vi "fgv_pc_clamp_result.vi"(7 "cmd":T6=enum."write_clamp_result", 8 "error in":errorcluster, 9 "clamp_roi_overlay-result_in":T3 {"ROI Descriptor out"."Contours"."Type" items=["No Selection", "Point", "Line", "Rectangle", "Oval", "Polygon", "Freehand Region", "Annulus", "Unused2", "Unused3", "Broken Line", "Freehand Line", "Rotated Rectangle"]}, 10 "mask_sum":cluster{u8, u8}, 11 "clamp result in":T5 {"clamp_result"."ROI Descriptor out"."Contours"."Type" items=["No Selection", "Point", "Line", "Rectangle", "Oval", "Polygon", "Freehand Region", "Annulus", "Unused2", "Unused3", "Broken Line", "Freehand Line", "Rotated Rectangle"]}) -> (0 "error out":errorcluster, 1 "clamp_roi_overlay-result_out":T2 {"ROI Descriptor out"."Contours"."Type" items=["No Selection", "Point", "Line", "Rectangle", "Oval", "Polygon", "Freehand Region", "Annulus", "Unused2", "Unused3", "Broken Line", "Freehand Line", "Rotated Rectangle"]}, 2 "mask_sum_out":cluster{u8, u8}, 3 "clamp result out":T4 {"clamp_result"."ROI Descriptor out"."Contours"."Type" items=["No Selection", "Point", "Line", "Rectangle", "Oval", "Polygon", "Freehand Region", "Annulus", "Unused2", "Unused3", "Broken Line", "Freehand Line", "Rotated Rectangle"]})   [LabVIEW 2019]
uses:
  Ctrl/clamp-result_cmd.ctl
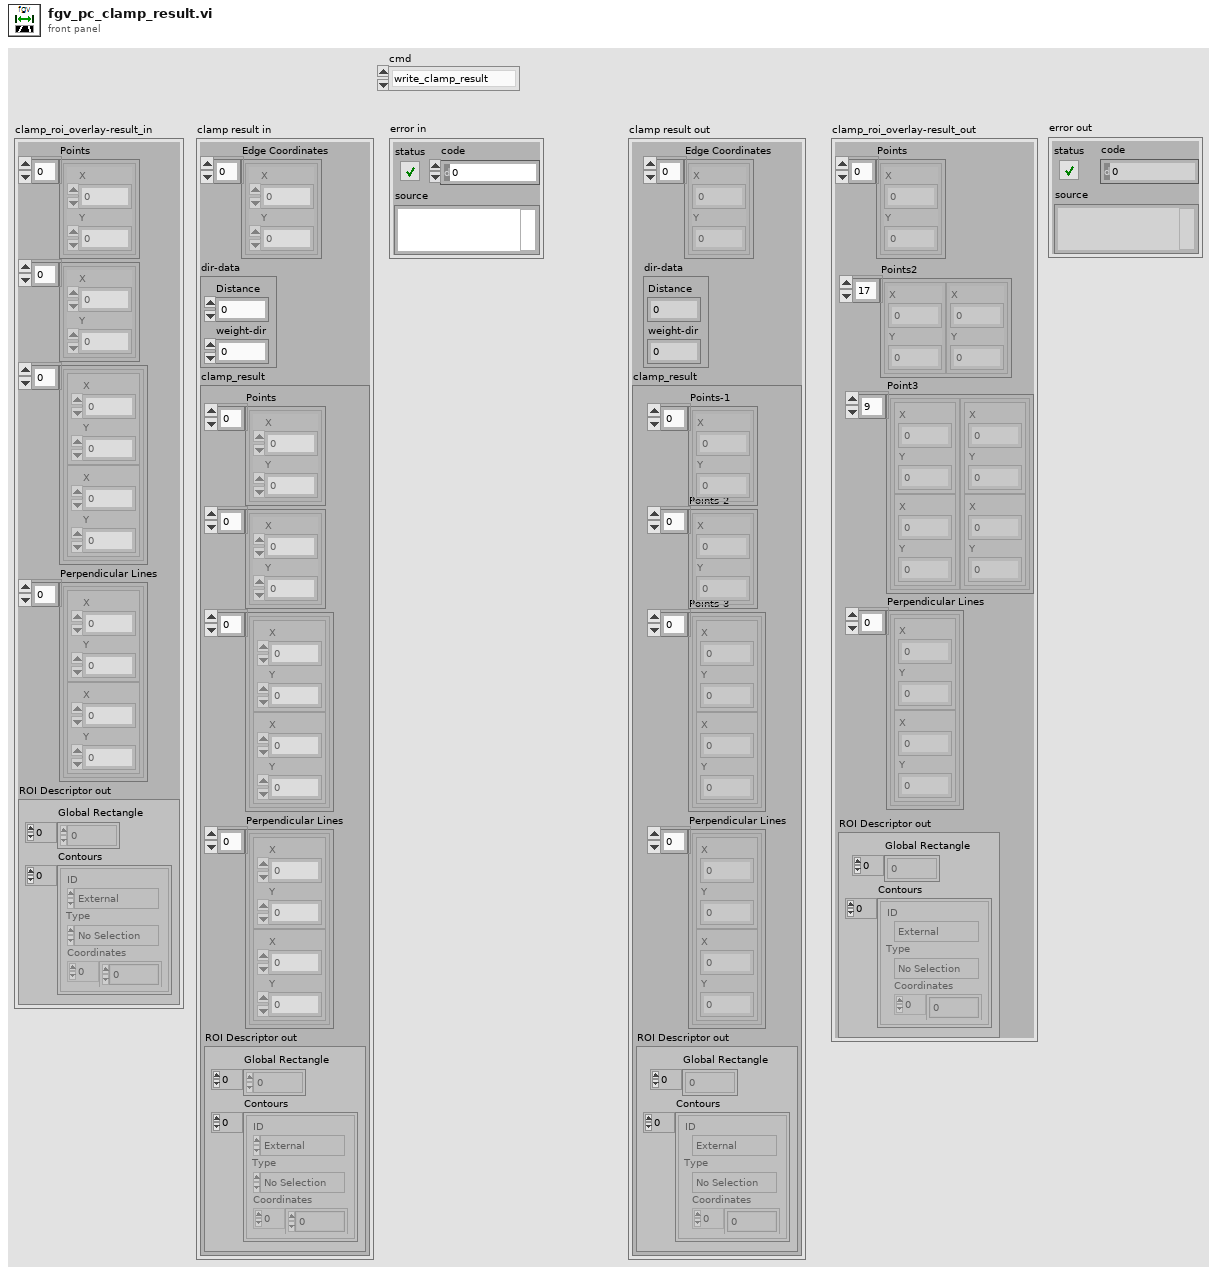
[diagram p1: front panel]
types:
  T1 = typedef "ROI Descriptor" = cluster{"Global Rectangle":i32[], "Contours":cluster{"ID":enum32{"External", "Internal"}, "Type":u32, "Coordinates":i32[]}[]}
  T2 = cluster{"Points":cluster{"X":sgl, "Y":sgl}[], "Points2":cluster{"X":sgl, "Y":sgl}[], "Point3":cluster{cluster{"X":sgl, "Y":sgl}, cluster{"X":sgl, "Y":sgl}}[], "Perpendicular Lines":cluster{cluster{"X":sgl, "Y":sgl}, cluster{"X":sgl, "Y":sgl}}[], "ROI Descriptor out":T1}
  T3 = cluster{"Points":cluster{"X":sgl, "Y":sgl}[], cluster{"X":sgl, "Y":sgl}[], cluster{cluster{"X":sgl, "Y":sgl}, cluster{"X":sgl, "Y":sgl}}[], "Perpendicular Lines":cluster{cluster{"X":sgl, "Y":sgl}, cluster{"X":sgl, "Y":sgl}}[], "ROI Descriptor out":T1}
  T4 = cluster{"Edge Coordinates":cluster{"X":sgl, "Y":sgl}[], "dir-data":cluster{"Distance":sgl, "weight-dir":dbl}, "clamp_result":cluster{"Points-1":cluster{"X":sgl, "Y":sgl}[], "Points-2":cluster{"X":sgl, "Y":sgl}[], "Points-3":cluster{cluster{"X":sgl, "Y":sgl}, cluster{"X":sgl, "Y":sgl}}[], "Perpendicular Lines":cluster{cluster{"X":sgl, "Y":sgl}, cluster{"X":sgl, "Y":sgl}}[], "ROI Descriptor out":T1}}
  T5 = cluster{"Edge Coordinates":cluster{"X":sgl, "Y":sgl}[], "dir-data":cluster{"Distance":sgl, "weight-dir":dbl}, "clamp_result":cluster{"Points":cluster{"X":sgl, "Y":sgl}[], cluster{"X":sgl, "Y":sgl}[], cluster{cluster{"X":sgl, "Y":sgl}, cluster{"X":sgl, "Y":sgl}}[], "Perpendicular Lines":cluster{cluster{"X":sgl, "Y":sgl}, cluster{"X":sgl, "Y":sgl}}[], "ROI Descriptor out":T1}}
  T6 = typedef "clamp-result_cmd.ctl" = enum16{"write_clamp_overlay-result", "write_center-distance", "write_clamp_result", "write_threshold_result", "read"}
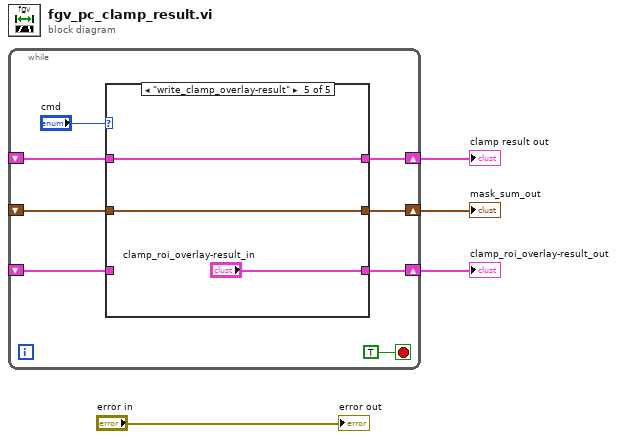
[diagram p0: block diagram]
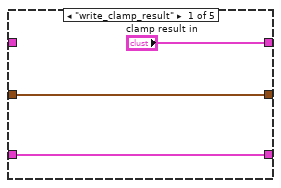
[diagram p2: hidden frame]
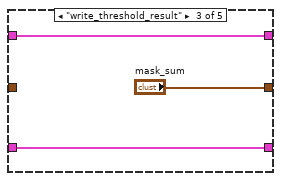
[diagram p4: hidden frame]
diagram:
  n1 = while {
    shift-right: [w8] -> w4
    shift-left: _ -> [w7]
    shift-right: [w10] -> w2
    shift-left: _ -> [w9]
    shift-right: [w6] -> w1
    shift-left: _ -> [w5]
    stop <- TRUE stop-if-true
    n2 = case shown="\"write_clamp_overlay-result\"" "cmd" {
      tunnel: ["clamp result in" w18 w21 w24 w27] -> w10
      tunnel: w9 -> [_ w18 w21 w24 w27]
      tunnel: [w15 w17 "mask_sum" w23 w26] -> w8
      tunnel: w7 -> [w15 w17 _ w23 w26]
      tunnel: [w13 w16 w19 w22 "clamp_roi_overlay-result_in"] -> w6
      tunnel: w5 -> [w13 w16 w19 w22 _]
      frame "write_clamp_result" {
      }
      frame "read", Default {
      }
      frame "write_threshold_result" {
      }
      frame "write_center-distance" {
      }
      frame "write_clamp_overlay-result" {
      }
    }
  }
  "mask_sum_out" <- w4
  "clamp result out" <- w2
  "clamp_roi_overlay-result_out" <- w1
  "error out" <- "error in"
